vi "dfd_LP to HP,BP,BS Mapping.vi"(1 "wo^2":dbl=0.9442719099991586 format="%.2f", 2 "filter type":T1(ring), 3 "LP poles/zeros":T2[](array[typedef])) -> (0 "transformed poles/zeros":T2[](array[typedef]))   [LabVIEW 2017, in "NI_DigFilter_Design.lvlib"]
uses:
  <vilib>/addons/Digital Filter Design/NI_DigFilter_Design.lvlib
  <vilib>/addons/Digital Filter Design/_Objects.llb/DFD Pole-Zero.ctl
  <vilib>/addons/Digital Filter Design/NI_DigFilterLicensed.lvlib
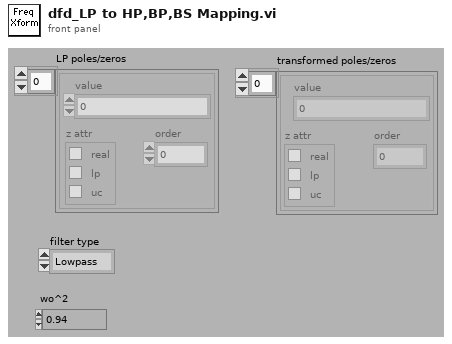
[diagram p1: front panel]
types:
  T1 = enum16{"Lowpass", "Highpass", "Bandpass", "Bandstop"}
  T2 = typedef "NI_DigFilterLicensed.lvlib/DFD Pole-Zero.ctl" = cluster{"value":cdb, "z attr":cluster{"real":bool, "lp":bool, "uc":bool}, "order":i32}
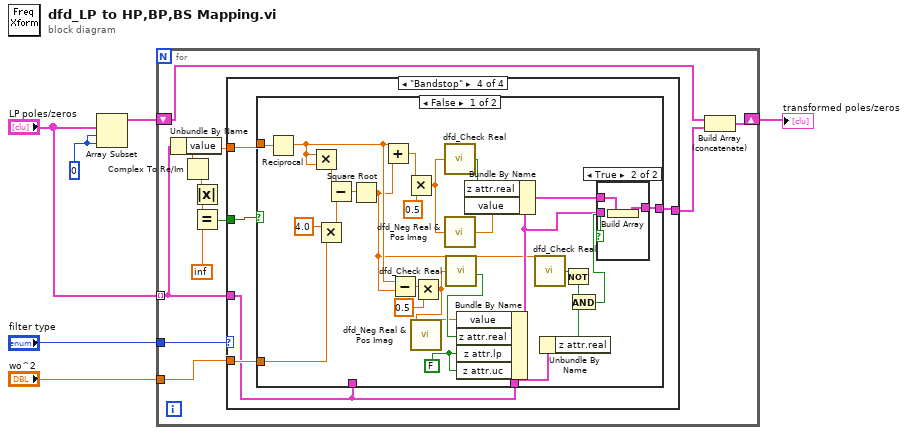
[diagram p0: block diagram]
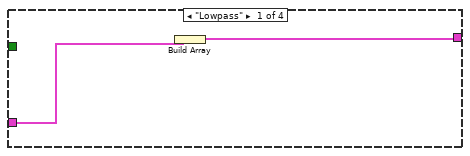
[diagram p2: hidden frame]
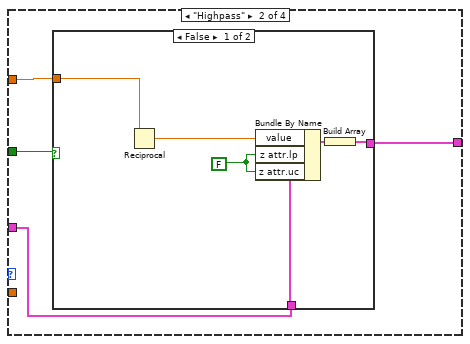
[diagram p3: hidden frame]
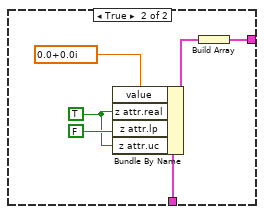
[diagram p4: hidden frame]
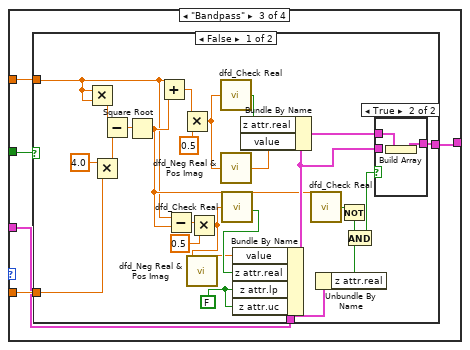
[diagram p5: hidden frame]
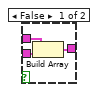
[diagram p6: hidden frame]
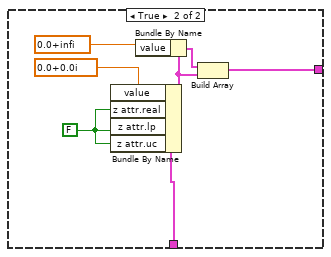
[diagram p7: hidden frame]
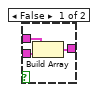
[diagram p8: hidden frame]
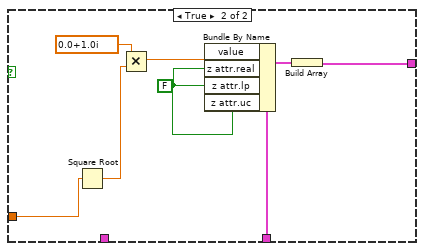
[diagram p9: hidden frame]
diagram:
  w2 = 0
  n1 = Array Subset(array="LP poles/zeros", index=w2, length=w2) -> (w4:T2[])
  n2 = for {
    tunnel: "LP poles/zeros" -> [w9] mode=indexing
    shift-right: [w7] -> w6
    shift-left: w4 -> [w17]
    tunnel: "filter type" -> [w15]
    tunnel: "wo^2" -> [w14]
    n3 = Unbundle By Name(w9) -> ("value"=w13:cdb)
    n4 = Complex To Re/Im(x + iy=w13) -> (y=w12:dbl)  [unwired: 1 out]
    n5 = Absolute Value(x=w12) -> (abs(x)=w10:dbl)
    n6 = Equal?(x=w10, y=inf) -> (x = y?=w8:bool)
    n7 = case shown="\"Bandstop\"" w15 {
      tunnel: [w19 w23 w36 w79] -> w16
      tunnel: w9 -> [w18 w22 w37 w80]
      tunnel: w14 -> [_ _ w38 w83]
      tunnel: w13 -> [_ w21 w39 w82]
      tunnel: w8 -> [_ w20 w40 w81]
      frame "Lowpass" {
        n8 = Build Array(w18) -> (w19:T2[])
      }
      frame "Highpass" {
        n9 = case shown="False" w20 {
          tunnel: [w29 w35] -> w23
          tunnel: w22 -> [w28 w34]
          tunnel: w21 -> [w24 _]
          frame False {
            w25 = FALSE
            n10 = Reciprocal(x=w24) -> (1/x=w26:cdb)
            n11 = Bundle By Name(cluster=w28, "value"=w26, "z attr.lp"=w25, "z attr.uc"=w25) -> (w27:T2)
            n12 = Build Array(w27) -> (w29:T2[])
          }
          frame True {
            w30 = TRUE
            n13 = Bundle By Name(cluster=w34, "value"=cdb 0.0+0.0i, "z attr.real"=w30, "z attr.lp"=FALSE, "z attr.uc"=w30) -> (w33:T2)
            n14 = Build Array(w33) -> (w35:T2[])
          }
        }
      }
      frame "Bandpass" {
        n15 = case shown="False" w40 {
          tunnel: [w45 w72] -> w36
          tunnel: w39 -> [w43 _]
          tunnel: w37 -> [w51 w73]
          tunnel: w38 -> [w42 _]
          frame False {
            w58 = FALSE
            n16 = Multiply(x=w43, y=w43) -> (x*y=w56:cdb)
            n17 = Multiply(x=4.0, y=w42) -> (x*y=w62:dbl)
            n18 = Subtract(x=w56, y=w62) -> (x-y=w60:cdb)
            n19 = Square Root(x=w60) -> (sqrt(x)=w44:cdb)
            n20 = Add(x=w43, y=w44) -> (x+y=w63:cdb)
            n21 = Subtract(x=w43, y=w44) -> (x-y=w66:cdb)
            n22 = Multiply(x=w63, y=0.5) -> (x*y=w54:cdb)
            n23 = Multiply(x=w66, y=0.5) -> (x*y=w52:cdb)
            n24 = call <vilib>:"dfd_Neg Real & Pos Imag.vi"("complex in"=w52) -> ("complex out"=w55:cdb)
            n25 = call <vilib>:"dfd_Check Real.vi"("complex"=w54) -> ("real?"=w59:bool)
            n26 = call <vilib>:"dfd_Neg Real & Pos Imag.vi"("complex in"=w54) -> ("complex out"=w53:cdb)
            n27 = call <vilib>:"dfd_Check Real.vi"("complex"=w52) -> ("real?"=w57:bool)
            n28 = Bundle By Name(cluster=w51, "value"=w55, "z attr.real"=w57, "z attr.lp"=w58, "z attr.uc"=w58) -> (w46:T2)
            n29 = Bundle By Name(cluster=w46, "z attr.real"=w59, "value"=w53) -> (w47:T2)
            n30 = call <vilib>:"dfd_Check Real.vi"("complex"=w44) -> ("real?"=w49:bool)
            n31 = Unbundle By Name(w51) -> ("z attr.real"=w50:bool)
            n32 = Not(x=w49) -> (.not. x?=w48:bool)
            n33 = And(x=w48, y=w50) -> (x .and. y?=w41:bool)
            n34 = case shown="True" w41 {
              tunnel: [w69 w71] -> w45
              tunnel: w47 -> [w68 w70]
              tunnel: w46 -> [w67 _]
              frame False {
                n35 = Build Array(w68, w67) -> (w69:T2[])
              }
              frame True {
                n36 = Build Array(w70) -> (w71:T2[])
              }
            }
          }
          frame True {
            w74 = FALSE
            n37 = Bundle By Name(cluster=w73, "value"=cdb 0.0+0.0i, "z attr.real"=w74, "z attr.lp"=w74, "z attr.uc"=w74) -> (w78:T2)
            n38 = Bundle By Name(cluster=w78, "value"=cdb 0.0+infi) -> (w75:T2)
            n39 = Build Array(w75, w78) -> (w72:T2[])
          }
        }
      }
      frame "Bandstop" {
        n40 = case shown="False" w81 {
          tunnel: [w85 w123] -> w79
          tunnel: w83 -> [w101 w117]
          tunnel: w82 -> [w102 _]
          tunnel: w80 -> [_ _]
          tunnel: w80 -> [w92 w116]
          frame False {
            w100 = FALSE
            n41 = Reciprocal(x=w102) -> (1/x=w97:cdb)
            n42 = Multiply(x=w97, y=w97) -> (x*y=w98:cdb)
            n43 = Multiply(x=4.0, y=w101) -> (x*y=w106:dbl)
            n44 = Subtract(x=w98, y=w106) -> (x-y=w104:cdb)
            n45 = Square Root(x=w104) -> (sqrt(x)=w84:cdb)
            n46 = Add(x=w97, y=w84) -> (x+y=w107:cdb)
            n47 = Subtract(x=w97, y=w84) -> (x-y=w110:cdb)
            n48 = Multiply(x=w107, y=0.5) -> (x*y=w95:cdb)
            n49 = Multiply(x=w110, y=0.5) -> (x*y=w93:cdb)
            n50 = call <vilib>:"dfd_Neg Real & Pos Imag.vi"("complex in"=w93) -> ("complex out"=w96:cdb)
            n51 = call <vilib>:"dfd_Check Real.vi"("complex"=w95) -> ("real?"=w103:bool)
            n52 = call <vilib>:"dfd_Neg Real & Pos Imag.vi"("complex in"=w95) -> ("complex out"=w94:cdb)
            n53 = call <vilib>:"dfd_Check Real.vi"("complex"=w93) -> ("real?"=w99:bool)
            n54 = Bundle By Name(cluster=w92, "value"=w96, "z attr.real"=w99, "z attr.lp"=w100, "z attr.uc"=w100) -> (w86:T2)
            n55 = Bundle By Name(cluster=w86, "z attr.real"=w103, "value"=w94) -> (w87:T2)
            n56 = call <vilib>:"dfd_Check Real.vi"("complex"=w84) -> ("real?"=w90:bool)
            n57 = Unbundle By Name(w92) -> ("z attr.real"=w91:bool)
            n58 = Not(x=w90) -> (.not. x?=w89:bool)
            n59 = And(x=w89, y=w91) -> (x .and. y?=w88:bool)
            n60 = case shown="True" w88 {
              tunnel: [w113 w115] -> w85
              tunnel: w87 -> [w112 w114]
              tunnel: w86 -> [w111 _]
              frame False {
                n61 = Build Array(w112, w111) -> (w113:T2[])
              }
              frame True {
                n62 = Build Array(w114) -> (w115:T2[])
              }
            }
          }
          frame True {
            w118 = FALSE
            n63 = Square Root(x=w117) -> (sqrt(x)=w122:dbl)
            n64 = Multiply(x=cdb 0.0+1.0i, y=w122) -> (x*y=w120:cdb)
            n65 = Bundle By Name(cluster=w116, "value"=w120, "z attr.real"=w118, "z attr.lp"=w118, "z attr.uc"=w118) -> (w119:T2)
            n66 = Build Array(w119) -> (w123:T2[])
          }
        }
      }
    }
    n67 = Build Array (concatenate)(w17, w16) -> (w7:T2[])
  }
  "transformed poles/zeros" <- w6
